vi "VerifyIpConnection.vi"(0 "IP_ADDR":string="169.254.70.191", 11 "error in (no error)":errorcluster, 12 "#OfAttempts":i32=5, 14 "Timeout (ms)":i32=5000) -> (1 "count":i32, 2 "Success":bool=TRUE, 3 "Ping Reply Info":T1={"Source Address"="169.254.70.191", "Bytes"=32, "Sequence"=0, "Time (ms)"=4, "Hops"=1, "TTL Returned"=255, "Status"="Reply from 169.254.70.191, Bytes=32, Sequence=0, Time=4ms, TTL=255 -> Hop(s)=1"} {"Sequence" format="%04x"}, 4 "ip_addr":string="169.254.70.191", 15 "error out":errorcluster)   [LabVIEW 2018]
uses:
  Ping Reply Info.ctl
panel:
  out "sec":dbl
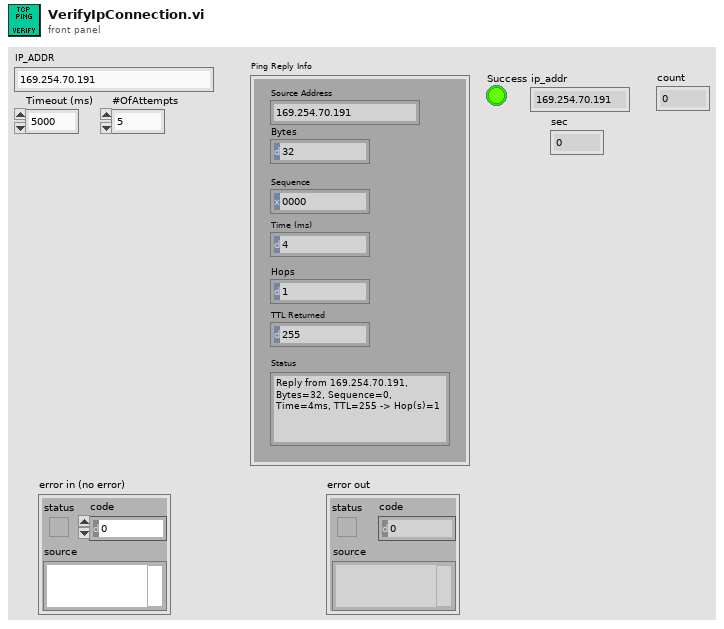
[diagram p1: front panel]
types:
  T1 = typedef "Ping Reply Info.ctl" = cluster{"Source Address":string, "Bytes":i32, "Sequence":u16, "Time (ms)":i32, "Hops":u8, "TTL Returned":u8, "Status":string}
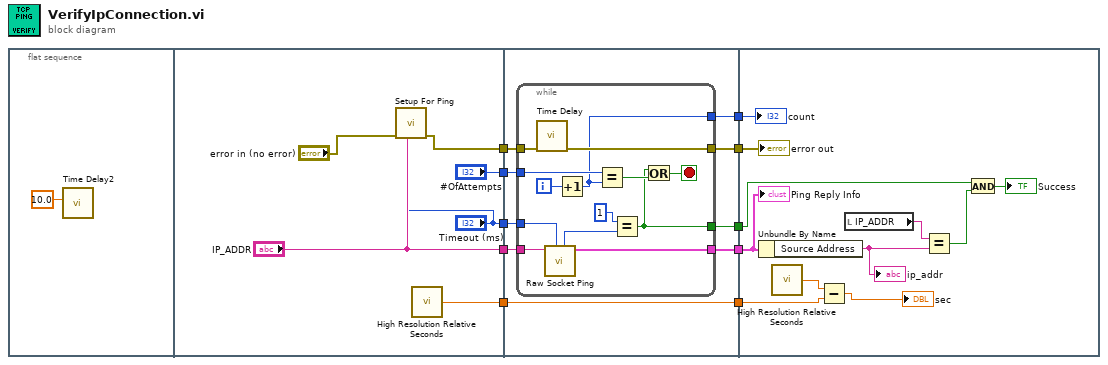
[diagram p0: block diagram]
diagram:
  n1 = flat-sequence {
    tunnel: ["IP_ADDR"] -> w7
    tunnel: ["Timeout (ms)"] -> w6
    tunnel: ["#OfAttempts"] -> w5
    tunnel: [w13] -> w4
    tunnel: [w16] -> w3
    tunnel: [w22] -> w10
    tunnel: [w21] -> w9
    tunnel: [w20] -> w8
    tunnel: w7 -> [w26]
    tunnel: w6 -> [w25]
    tunnel: w5 -> [w24]
    tunnel: w4 -> [w23]
    tunnel: w3 -> [w19]
    tunnel: [w19] -> w2
    tunnel: [w18] -> w1
    tunnel: w10 -> [w50]
    tunnel: w9 -> [w48]
    tunnel: w8 -> [w44]
    tunnel: w2 -> [w42]
    tunnel: w1 -> [w40]
    frame #0 {
      n2 = call "Time Delay2"("Delay Time (s)"=10.0) -> ()  [unwired: 10 in, 1 out]
    }
    frame #1 {
      n3 = call "Setup For Ping.vi"("Timeout (ms)"="Timeout (ms)", "Host to Ping"="IP_ADDR", "Error In"="error in (no error)") -> ("Error Out"=w13:errorcluster)  [unwired: 6 in, 2 out]
      n4 = call <vilib>:"High Resolution Relative Seconds.vi"() -> ("relative seconds"=w16:dbl)
    }
    frame #2 {
      n5 = while {
        tunnel: w26 -> [w39]
        tunnel: w25 -> [w38]
        tunnel: [w37] -> w22
        tunnel: w24 -> [w32]
        tunnel: [w30] -> w21
        tunnel: w23 -> [w29]
        tunnel: [w28] -> w20
        tunnel: [w27] -> w18
        i -> [w33]
        stop <- w36 stop-if-true
        n6 = call "Time Delay"("error in (no error)"=w29) -> ("error out"=w28:errorcluster)  [unwired: 10 in]
        n7 = call "Raw Socket Ping.vi"("Host to Ping"=w39, "Timeout (ms)"=w38) -> ("RxCount"=w35:i32, "Ping Reply Info"=w37:T1)  [unwired: 6 in, 1 out]
        n8 = Increment(x=w33) -> (x+1=w27:i32)
        n9 = Equal?(x=w32, y=w27) -> (x = y?=w31:bool)
        n10 = Equal?(x=1, y=w35) -> (x = y?=w30:bool)
        n11 = Or(x=w30, y=w31) -> (x .or. y?=w36:bool)
      }
    }
    frame #3 {
      n12 = Unbundle By Name(w50) -> ("Source Address"=w47:string)
      "ip_addr" <- w47
      n13 = call <vilib>:"High Resolution Relative Seconds.vi"() -> ("relative seconds"=w43:dbl)
      n14 = Subtract(x=w43, y=w42) -> (x-y=→"sec":dbl)
      n15 = local read "IP_ADDR"() -> (w46:string)
      n16 = Equal?(x=w46, y=w47) -> (x = y?=w45:bool)
      n17 = And(x=w48, y=w45) -> (x .and. y?=→"Success":bool)
      "Ping Reply Info" <- w50
      "error out" <- w44
      "count" <- w40
    }
  }
